vi "data manip.vi"(9 "Points to be deleted":i32, 10 "Skip points":bool, 11 "UDP Data Array (in)":cluster{"Array":string[], "Numeric":i32}[](array[cluster])) -> (2 "points num array":i32[](array[numeric]), 3 "UDP Data Array (Out)":cluster{"Array":string[], "Numeric":i32}[](array[cluster]))   [LabVIEW 2021]
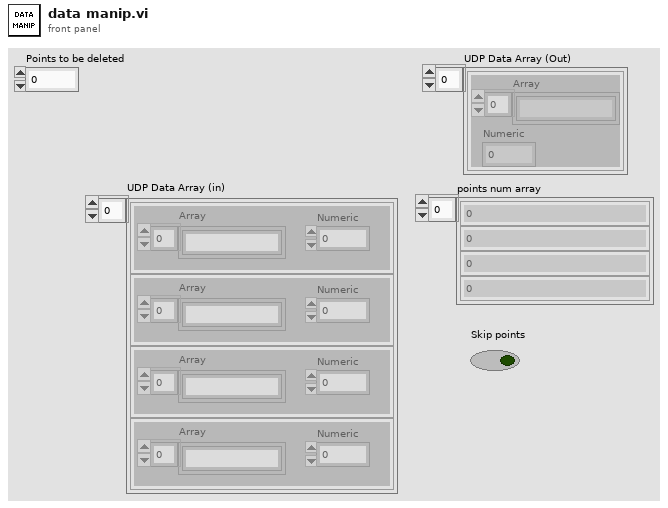
[diagram p1: front panel]
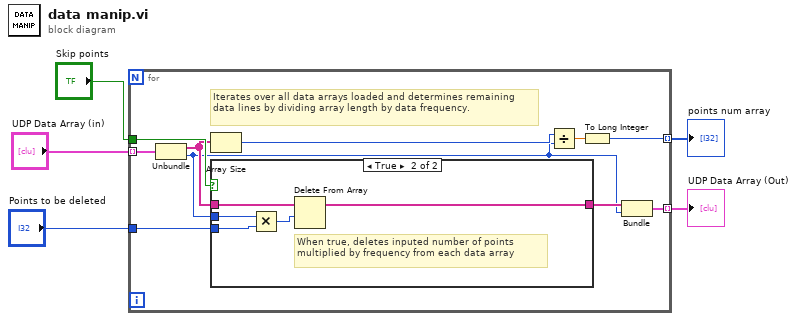
[diagram p0: block diagram]
diagram:
  n1 = for {
    tunnel: "UDP Data Array (in)" -> [w15] mode=indexing
    tunnel: [w12] -> w4 mode=indexing
    tunnel: "Skip points" -> [w11]
    tunnel: [w8] -> w3 mode=indexing
    tunnel: "Points to be deleted" -> [w6]
    # "Iterates over all data arrays loaded and determines remaining data lines by dividing array length by data frequency."
    n2 = Unbundle(w15) -> ("Array"=w10:string[], "Numeric"=w7:i32)
    n3 = Array Size(array=w10) -> (size(s)=w14:i32)
    n4 = case shown="True" w11 {
      tunnel: w10 -> [w16 w21]
      tunnel: [w16 w20] -> w9
      tunnel: w7 -> [_ w18]
      tunnel: w6 -> [_ w17]
      frame False {
      }
      frame True {
        # "When true, deletes inputed number of points multiplied by frequency from each data array"
        n5 = Multiply(x=w18, y=w17) -> (x*y=w19:i32)
        n6 = Delete From Array(array=w21, length=w19) -> (array with subset deleted=w20:string[])  [unwired: 1 in, 1 out]
      }
    }
    n7 = Divide(x=w14, y=w7) -> (x/y=w13:dbl)
    n8 = To Long Integer(number=w13) -> (32bit integer=w12:i32)
    n9 = Bundle("Array"=w9, "Numeric"=w7) -> (w8:cluster{"Array":string[], "Numeric":i32})  [unwired: 1 in]
  }
  "points num array" <- w4
  "UDP Data Array (Out)" <- w3
